vi "Initialize.vi"(8 "error in (no error)":errorcluster, 9 "Timeout [ms] (5000)":i32=5000, 10 "Connection":refnum<class "Connection.lvclass">, 11 "Connection in":refnum<class "Connection.lvclass">) -> (0 "error out":errorcluster, 3 "Connection out":refnum<class "Connection.lvclass">)   [LabVIEW 2022 SP3, in "Connection.lvlib" / "Connection.lvclass"]
uses:
  Connection.lvclass
  Connection.lvclass/Connection.ctl
  _State.ctl
  <vilib>/ActorFramework/Actor/Actor.lvclass
  Connection Messages/WaitForData Msg/WaitForData Msg.lvclass
  C:/Program Files (x86)/National Instruments/LabVIEW 2022/vi.lib/ActorFramework/Actor/Actor.lvclass
  TcpSocket/Source/TcpSocket/Connection/Connection.lvclass
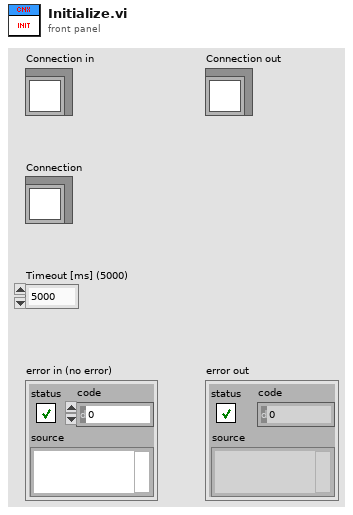
[diagram p1: front panel]
types:
  T1 = typedef "Connection.lvlib/Connection.lvclass/_State.ctl" = enum16{"WaitForInit", "Active", "Dying"}
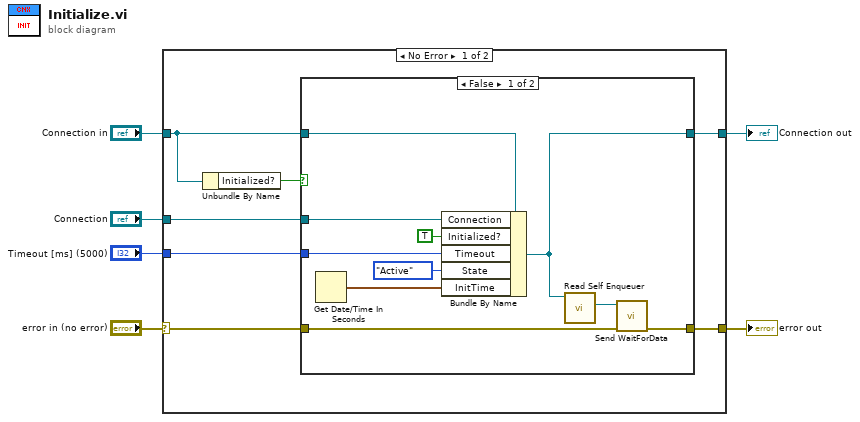
[diagram p0: block diagram]
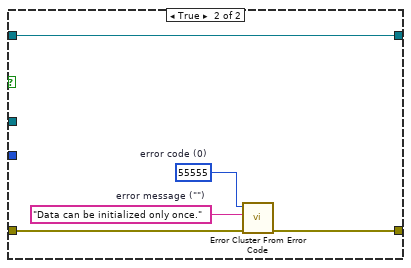
[diagram p2: hidden frame]
diagram:
  n1 = case shown="No Error" "error in (no error)" {
    selector: "error in (no error)" -> [w9 w30]
    tunnel: [w8 w30] -> w5
    tunnel: [w12 w29] -> w3
    tunnel: "Connection in" -> [w11 w29]
    tunnel: "Connection" -> [w13 _]
    tunnel: "Timeout [ms] (5000)" -> [w7 _]
    frame No Error {
      n2 = Unbundle By Name(w11) -> ("Initialized?"=w10:bool)
      n3 = case shown="False" w10 {
        tunnel: w13 -> [w23 _]
        tunnel: [w17 w28] -> w12
        tunnel: w11 -> [w21 w28]
        tunnel: w9 -> [w14 w27]
        tunnel: [w15 w26] -> w8
        tunnel: w7 -> [w20 _]
        frame False {
          n4 = Get Date/Time In Seconds() -> (seconds since 1Jan1904=w18:timestamp)
          n5 = Bundle By Name(cluster=w21, "Connection"=w23, "Initialized?"=TRUE, "Timeout"=w20, "State"=_State."Active", "InitTime"=w18) -> (w17:refnum<class "Connection.lvclass">)
          n6 = call <vilib>:"Read Self Enqueuer.vi"("Actor"=w17) -> ("Self Enqueuer"=w16:refnum<class "Message Enqueuer.lvclass">)  [unwired: 10 in]
          n7 = call "Send WaitForData.vi"("error in (no error)"=w14, "Message Enqueuer"=w16) -> ("error out"=w15:errorcluster)  [unwired: 8 in, 1 out]
        }
        frame True {
          w24 = 55555  # error code (0)
          w25 = "Data can be initialized only once."  # error message ("")
          n8 = call <vilib>:"Error Cluster From Error Code.vi"("error in (no error)"=w27, "error message (\"\")"=w25, "error code (0)"=w24) -> ("error out"=w26:errorcluster)  [unwired: 6 in]
        }
      }
    }
    frame Error {
    }
  }
  "error out" <- w5
  "Connection out" <- w3
